vi "OP300ZP_ATEQ.vi"(8 "entrée d'erreur (pas d'erreur)":errorcluster) -> (0 "sortie d'erreur":errorcluster, 2 "Valeur d'étanchéité":dbl, 3 "Case à cocher":bool)   [LabVIEW 2020]
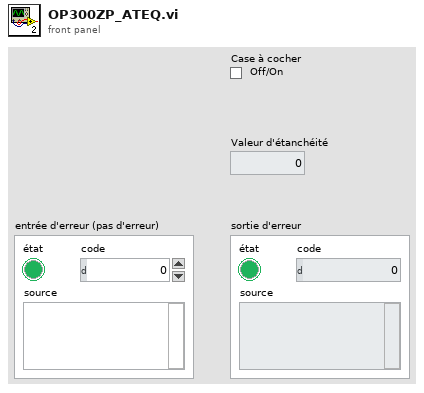
[diagram p1: front panel]
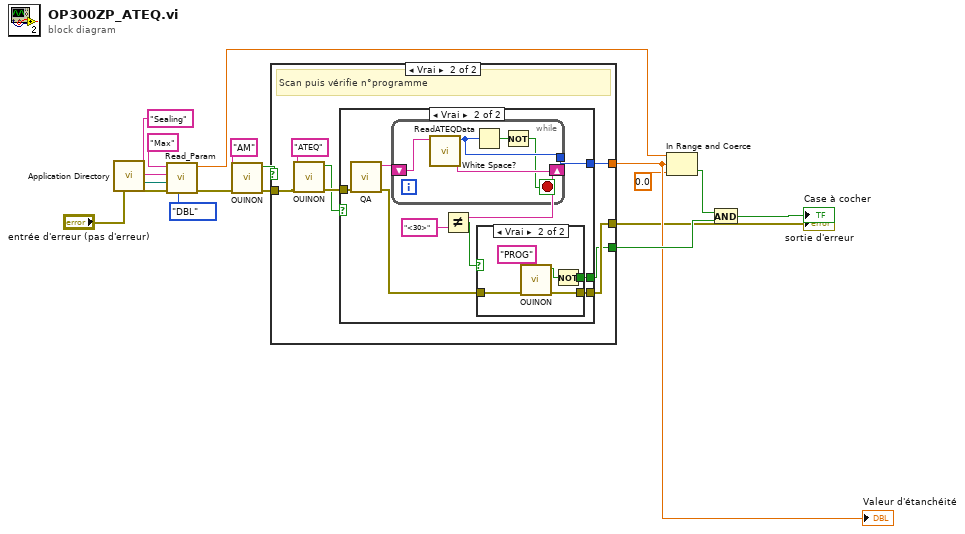
[diagram p0: block diagram]
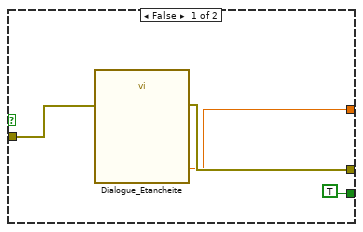
[diagram p2: hidden frame]
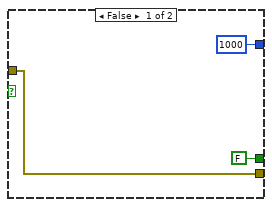
[diagram p3: hidden frame]
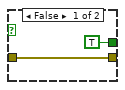
[diagram p4: hidden frame]
diagram:
  n1 = call <vilib>:"Application Directory.vi"() -> ("Application Directory"=w1:path)
  n2 = call "Read_Param.vi"("Énum"=enum16{"STR", "DBL", "U32"}."DBL", "errin"="entrée d'erreur (pas d'erreur)", "pathin"=w1, "section"="Sealing", "key"="Max") -> ("error out"=w14:errorcluster, "dbl"=w6:dbl)  [unwired: 2 in, 3 out]
  n3 = call <vilib>:"OUINON.vi"("errin"=w14, "image"="AM" ("IN")) -> ("error out"=w16:errorcluster, "OUI/NON"=w15:bool)  [unwired: 8 in]
  n4 = case shown="Vrai" w15 {
    tunnel: [w19 w27] -> w8
    tunnel: [w20 w26] -> w7
    tunnel: [TRUE w25] -> w10
    tunnel: w16 -> [w17 w23]
    frame False {
      n5 = call "Dialogue_Etancheite.vi"("error in (no error)"=w17) -> ("Valeur d'étanchéité"=w19:dbl, "error out"=w20:errorcluster)  [unwired: 16 in, 1 out]
    }
    frame True {
      # "Scan puis vérifie n°programme"
      n6 = call <vilib>:"OUINON.vi"("errin"=w23, "image"="ATEQ" ("IN")) -> ("error out"=w22:errorcluster, "OUI/NON"=w21:bool)  [unwired: 8 in]
      n7 = case shown="Vrai" w21 {
        tunnel: [1000 ("Valeur") w39] -> w27
        tunnel: [w30 w36] -> w26
        tunnel: [FALSE w35] -> w25
        tunnel: w22 -> [w30 w31]
        frame False {
        }
        frame True {
          n8 = call "QA.vi"("ERRIN"=w31) -> ("ERROUT"=w37:errorcluster, "DATA OUT"=w38:string)  [unwired: 9 in]
          n9 = while {
            tunnel: [w44] -> w39
            shift-right: [w42] -> w34
            shift-left: w38 -> [w43]
            stop <- w40 stop-if-true
            n10 = call "ReadATEQData.vi"("Chaîne"=w43) -> ("Prg number"=w42:string, "Valeur"=w44:i32)  [unwired: 7 in, 2 out]
            n11 = White Space?(1:w44) -> (0:w41:bool)
            n12 = Not(x=w41) -> (.not. x?=w40:bool)
          }
          n13 = Not Equal?(x=w34, y="<30>") -> (x != y?=w32:bool)
          n14 = case shown="Vrai" w32 {
            tunnel: w37 -> [w45 w50]
            tunnel: [w45 w49] -> w36
            tunnel: [TRUE w47] -> w35
            frame False {
            }
            frame True {
              n15 = call <vilib>:"OUINON.vi"("errin"=w50, "image"="PROG" ("IN")) -> ("error out"=w49:errorcluster, "OUI/NON"=w48:bool)  [unwired: 8 in]
              n16 = Not(x=w48) -> (.not. x?=w47:bool)
            }
          }
        }
      }
    }
  }
  "Valeur d'étanchéité" <- w8
  "sortie d'erreur" <- w7
  n17 = In Range and Coerce ("Dans la gamme")(upper limit=w6, x=w8, lower limit=0.0 ("limite inférieure")) -> (In Range?=w9:bool)  [unwired: 1 out]
  n18 = And(x=w9, y=w10) -> (x .and. y?=→"Case à cocher":bool)
